vi "Beam Permit Main.vi"() -> ()   [LabVIEW 2019]
panel:
  in  "Warning sound":bool
  in  "Bypass the FMag status":bool
  out "Beam Permit":bool
  in  "Force ON Beam permit":bool
  in  "Force OFF Beam permit":bool
  out "Beam permit status":string
  out "Warning play time":u32
  out "TCP":bool
  in  "Exit VI":bool
  out "Fmag Low Current attemps":i32
  out "Error status":T1(ring)
  out "FMag monitor":u8(slide) scale=0.0..25.0
  out "chart_temp 2":waveform(dbl)[](graph)=[{"t0"=timestamp(3772890114.31303 s since 1904-01-01), "dt"=1.0, "Y"=[0.8687935985565186]}, {"t0"=timestamp(3772890114.31303 s since 1904-01-01), "dt"=1.0, "Y"=[86.87935985565186]}, {"t0"=timestamp(3772890114.31303 s since 1904-01-01), "dt"=1.0, "Y"=[30.48853325313992]}, {"t0"=timestamp(3772890114.31303 s since 1904-01-01), "dt"=1.0, "Y"=[303.6385332531399]}] caption="FMag Current"
  out "FMag Current (A)":dbl
  out "error out":errorcluster
  out "Target  Ready":bool
  out "FMag Ready":bool
  # "SpinQuest Beam Permit Signaller"
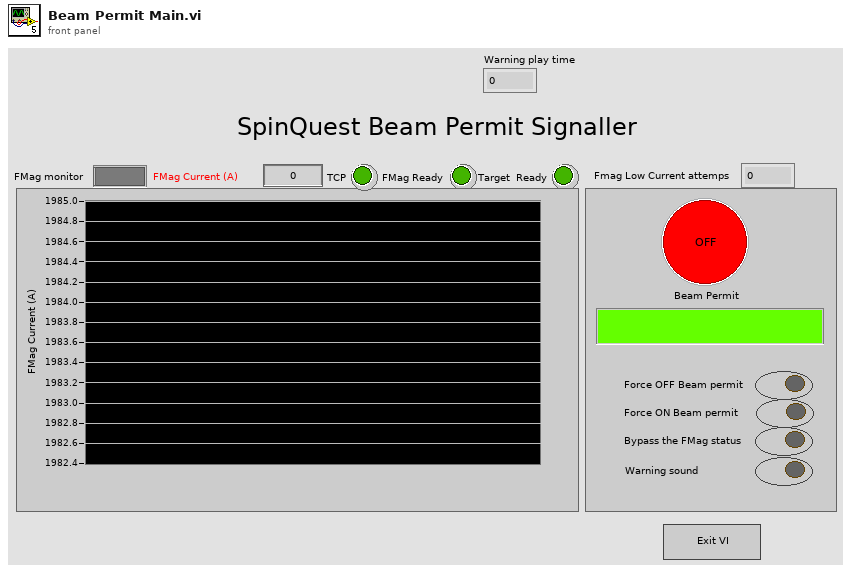
[diagram p1: front panel]
types:
  T1 = enum16{"No Error", "Les than 1800", "Les than 1500", "Les than 200", "Read out Error"}
  T2 = typedef "Sound Output Task ID.ctl" = u32
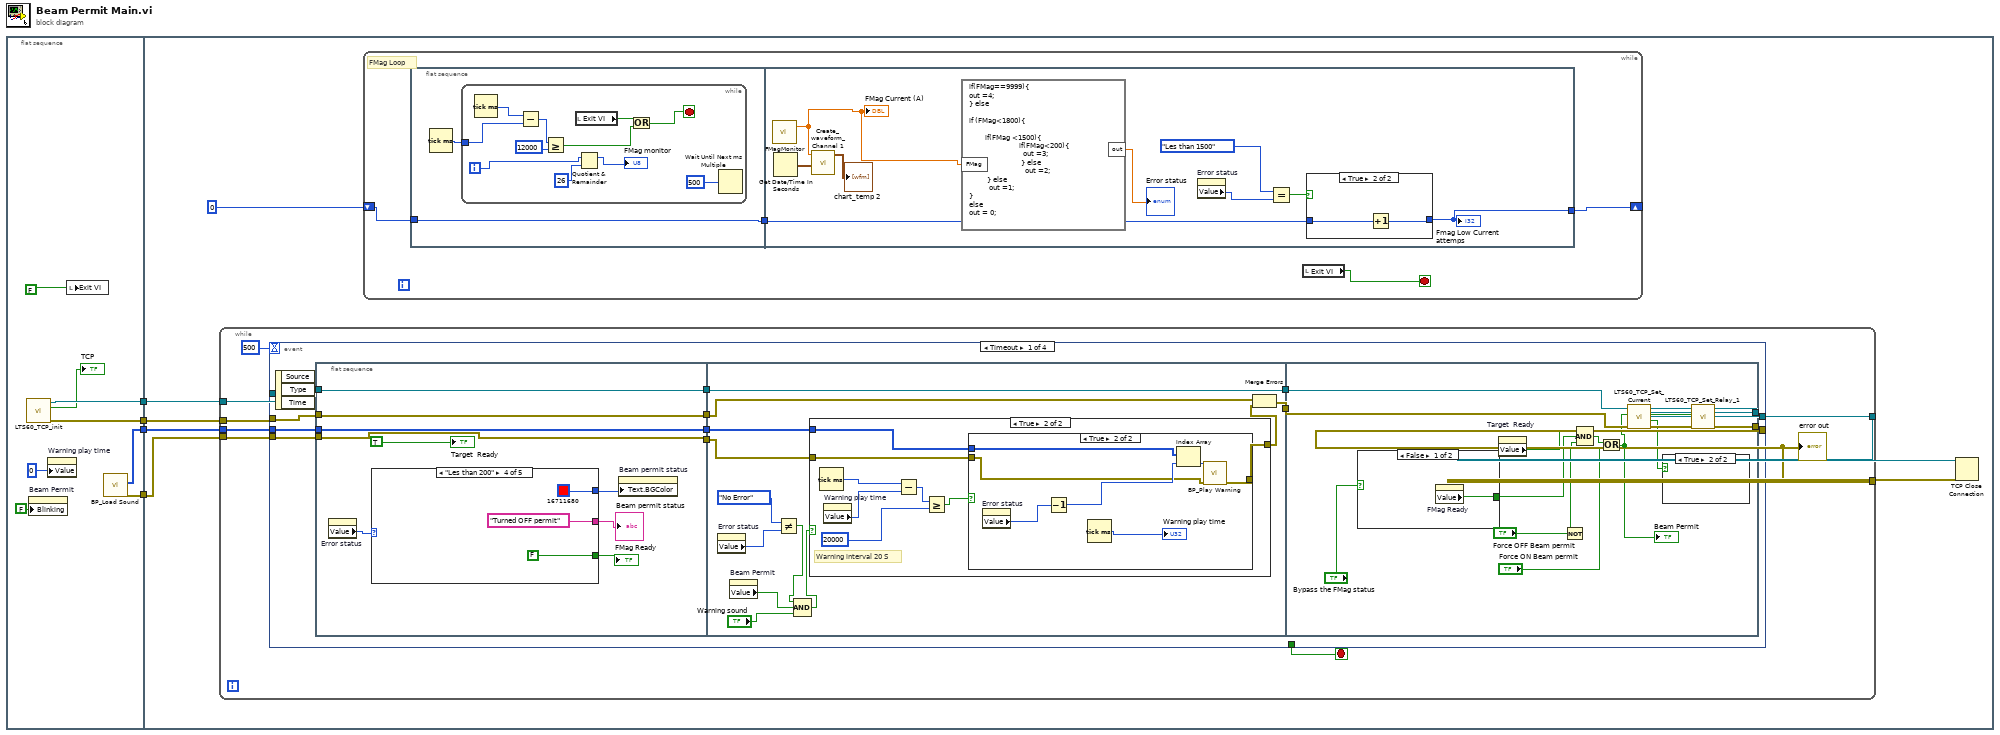
[diagram p0: block diagram]
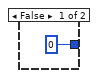
[diagram p2: hidden frame]
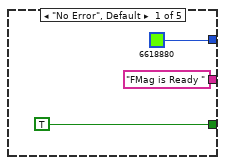
[diagram p3: hidden frame]
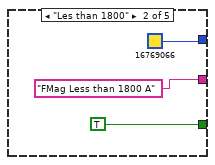
[diagram p4: hidden frame]
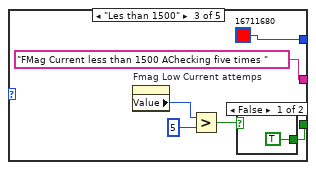
[diagram p5: hidden frame]
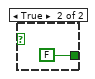
[diagram p6: hidden frame]
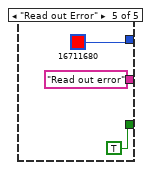
[diagram p7: hidden frame]
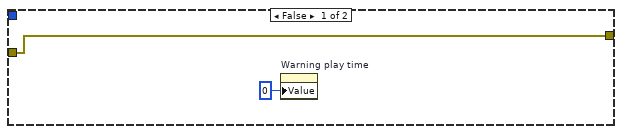
[diagram p8: hidden frame]
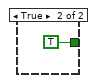
[diagram p11: hidden frame]
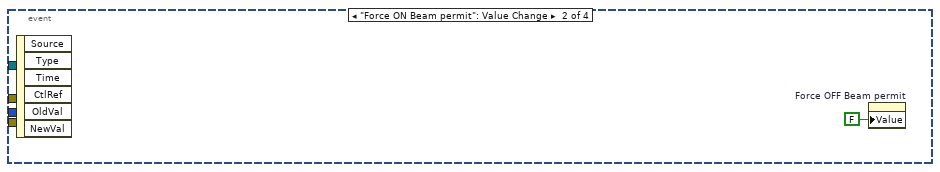
[diagram p12: hidden frame]
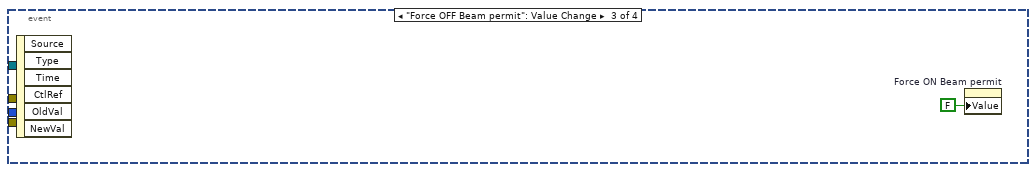
[diagram p13: hidden frame]
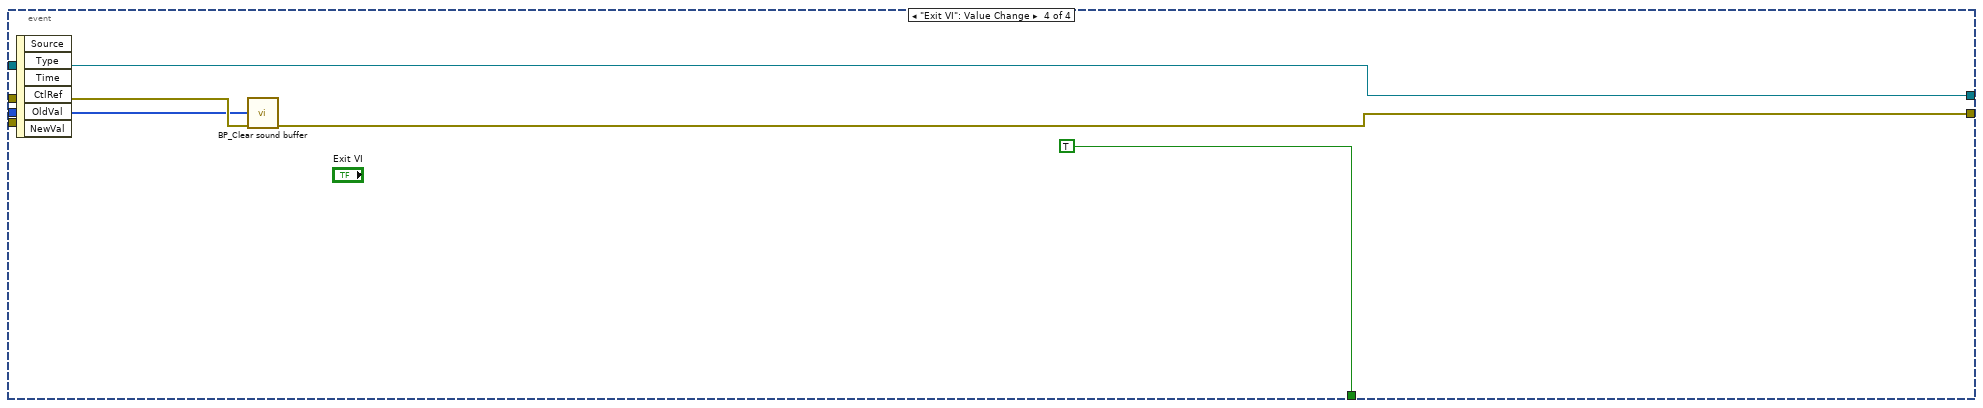
[diagram p14: hidden frame]
diagram:
  n1 = flat-sequence {
    tunnel: [w12] -> w4
    tunnel: [w11] -> w3
    tunnel: [w7] -> w2
    tunnel: [w5] -> w1
    tunnel: w4 -> [w14]
    tunnel: w3 -> [w17]
    tunnel: w2 -> [w15]
    tunnel: w1 -> [w13]
    frame #0 {
      n2 = call "LTS60_TCP_init.vi"() -> ("error out"=w12:errorcluster, "TCP Connected"=→"TCP":bool, "connection ID out"=w11:refnum<k5>)  [unwired: 9 in]
      n3 = property on="Beam Permit" class="Bool (strict)"("Blinking"=FALSE) -> ()  [unwired: 2 in, 2 out]
      n4 = property on="Warning play time" class="DigNum (strict)"("Value"=u32 0 ("Warning play time")) -> ()  [unwired: 2 in, 2 out]
      n5 = local write "Exit VI"(FALSE ("Exit VI")) -> ()
      n6 = call "BP_Load Sound.vi"() -> ("error out"=w5:errorcluster, "Sound Array"=w7:T2[])  [unwired: 9 in, 1 out]
    }
    frame #1 {
      n7 = while {
        tunnel: [w54] -> w18
        tunnel: [w53] -> w19
        tunnel: w14 -> [w52]
        tunnel: w17 -> [w51]
        tunnel: w15 -> [w50]
        tunnel: w13 -> [w49]
        stop <- w56 stop-if-true
        n8 = event shown="[0] Timeout" {
          selector: _ -> [_ _ _ _]
          dyn-events: _ -> [_ _ _ _]
          timeout: 500 -> [_ _ _ _]
          tunnel: [_ _ _ TRUE] -> w56
          tunnel: [w68 _ _ w148] -> w54
          tunnel: [w67 _ _ w151] -> w53
          tunnel: w51 -> [w65 _ _ w151]
          tunnel: w52 -> [w62 _ _ w150]
          tunnel: w50 -> [w60 _ _ w149]
          tunnel: w49 -> [w57 _ _ _]
          event Timeout {
            n9 = event-data() -> ()  [unwired: 1 in, 3 out]
            n10 = flat-sequence {
              tunnel: [w76] -> w66
              tunnel: w65 -> [w76]
              tunnel: [w75] -> w63
              tunnel: w62 -> [w75]
              tunnel: w60 -> [w71]
              tunnel: [w71] -> w59
              tunnel: [w70] -> w58
              tunnel: w57 -> [w70]
              tunnel: w66 -> [w109]
              tunnel: [w109] -> w64
              tunnel: w63 -> [w98]
              tunnel: [w100] -> w61
              tunnel: w59 -> [w106]
              tunnel: w58 -> [w101]
              tunnel: [w139] -> w68
              tunnel: [w138] -> w67
              tunnel: w64 -> [w142]
              tunnel: w61 -> [w136]
              frame #0 {
                n11 = property on="Error status" class="Enum (strict)"() -> ("Value"=w72:T1)  [unwired: 2 in, 2 out]
                n12 = case shown="\"Les than 200\"" w72 {
                  tunnel: [TRUE ("Magnet status") TRUE ("Magnet status") w89 FALSE ("Magnet status") TRUE ("Magnet status")] -> w73
                  tunnel: ["FMag is Ready " ("Beam permit status") "FMag Less than 1800 A" ("Beam permit status") "FMag Current less than 1500 AChecking five times " ("Beam permit status") "Turned OFF permit" ("Beam permit status") "Read out error" ("Beam permit status")] -> w74
                  tunnel: [u32 6618880 ("Text.Text Colors:BG Color") u32 16769066 ("Text.Text Colors:BG Color") u32 16711680 ("Text.Text Colors:BG Color") u32 16711680 ("Text.Text Colors:BG Color") u32 16711680 ("Text.Text Colors:BG Color")] -> w69
                  frame "No Error", Default {
                  }
                  frame "Les than 1800" {
                  }
                  frame "Les than 1500" {
                    n13 = property on="Fmag Low Current attemps" class="DigNum (strict)"() -> ("Value"=w88:i32)  [unwired: 2 in, 2 out]
                    n14 = Greater?(x=w88, y=5) -> (0:w86:bool)
                    n15 = case shown="False" w86 {
                      tunnel: [TRUE ("Magnet status") FALSE ("Magnet status")] -> w89
                      frame False {
                      }
                      frame True {
                      }
                    }
                  }
                  frame "Les than 200" {
                  }
                  frame "Read out Error" {
                  }
                }
                "FMag Ready" <- w73
                "Beam permit status" <- w74
                n16 = property on="Beam permit status" class="Str"("Text.BGColor"=w69) -> ()  [unwired: 2 in, 2 out]
                "Target  Ready" <- TRUE ("Target  status")
              }
              frame #1 {
                n17 = property on="Error status" class="Enum (strict)"() -> ("Value"=w108:T1)  [unwired: 2 in, 2 out]
                n18 = property on="Beam Permit" class="Bool (strict)"() -> ("Value"=w104:bool)  [unwired: 2 in, 2 out]
                n19 = Not Equal?(x=T1."No Error", y=w108) -> (x != y?=w103:bool)
                n20 = Compound Arithmetic op=AND(w103, w104, "Warning sound") -> (w102:bool)
                n21 = case shown="True" w102 {
                  tunnel: w106 -> [_ w114]
                  tunnel: [w110 w113] -> w99
                  tunnel: w101 -> [w110 w112]
                  frame False {
                    n22 = property on="Warning play time" class="DigNum (strict)"("Value"=u32 0 ("Warning play time")) -> ()  [unwired: 2 in, 2 out]
                  }
                  frame True {
                    # "Warning interval 20 S"
                    n23 = Tick Count (ms)() -> (millisecond timer value=w119:u32)
                    n24 = property on="Warning play time" class="DigNum (strict)"() -> ("Value"=w118:u32)  [unwired: 2 in, 2 out]
                    n25 = Subtract(x=w119, y=w118) -> (x-y=w117:u32)
                    n26 = Greater Or Equal?(x=w117, y=u32 20000) -> (x >= y?=w115:bool)
                    n27 = case shown="True" w115 {
                      tunnel: w114 -> [_ w125]
                      tunnel: [w120 w122] -> w113
                      tunnel: w112 -> [w120 w121]
                      frame False {
                      }
                      frame True {
                        n28 = property on="Error status" class="Enum (strict)"() -> ("Value"=w127:T1)  [unwired: 2 in, 2 out]
                        n29 = Decrement(x=w127) -> (x-1=w124:T1)
                        n30 = Tick Count (ms)() -> (millisecond timer value=→"Warning play time":u32)
                        n31 = Index Array(array=w125, index=w124) -> (element=w123:T2)
                        n32 = call "BP_Play Warning.vi"("error in (no error)"=w121, "task ID"=w123) -> ("error out"=w122:errorcluster)  [unwired: 8 in, 1 out]
                      }
                    }
                  }
                }
                n33 = Merge Errors(w98, w99) -> (w100:errorcluster)
              }
              frame #2 {
                n34 = case shown="False" "Bypass the FMag status" {
                  tunnel: [w144 TRUE ("Value")] -> w132
                  frame False {
                    n35 = property on="FMag Ready" class="Bool (strict)"() -> ("Value"=w144:bool)  [unwired: 2 in, 2 out]
                  }
                  frame True {
                  }
                }
                n36 = property on="Target  Ready" class="Bool (strict)"() -> ("Value"=w143:bool)  [unwired: 2 in, 2 out]
                n37 = Not(x="Force OFF Beam permit") -> (.not. x?=w131:bool)
                n38 = Compound Arithmetic op=AND(w143, w132, w131) -> (w134:bool)
                n39 = Or(x=w134, y="Force ON Beam permit") -> (x .or. y?=w129:bool)
                "Beam Permit" <- w129
                n40 = call "LTS60_TCP_Set_Current.vi"("error in (no error)"=w136, "Beam"=w129, "connection ID"=w142) -> ("error out"=w140:errorcluster, "Acknowladged"=w128:bool, "Beam out"=w137:bool, "connection ID out"=w141:refnum<k5>)  [unwired: 5 in]
                n41 = case shown="True" w128 {
                  frame False {
                  }
                  frame True {
                  }
                }
                n42 = call "LTS60_TCP_Set_Relay_1.vi"("error in (no error)"=w140, "Beam"=w137, "connection ID"=w141) -> ("error out"=w139:errorcluster, "connection ID out"=w138:refnum<k5>)  [unwired: 6 in, 1 out]
              }
            }
          }
          event "Force ON Beam permit": Value Change {
            n43 = event-data() -> ()  [unwired: 1 in, 6 out]
            n44 = property on="Force OFF Beam permit" class="Bool (strict)"("Value"=FALSE ("Force OFF Beam permit")) -> ()  [unwired: 2 in, 2 out]
          }
          event "Force OFF Beam permit": Value Change {
            n45 = event-data() -> ()  [unwired: 1 in, 6 out]
            n46 = property on="Force ON Beam permit" class="Bool (strict)"("Value"=FALSE ("Force ON Beam permit")) -> ()  [unwired: 2 in, 2 out]
          }
          event "Exit VI": Value Change {
            n47 = event-data() -> ()  [unwired: 1 in, 6 out]
            n48 = call "BP_Clear sound buffer.vi"("error in (no error)"=w150, "array"=w149) -> ("error out"=w148:errorcluster)  [unwired: 9 in]
          }
        }
        "error out" <- w54
      }
      n49 = while {
        shift-right: [w21] -> _
        shift-left: 0 ("Low Fmag attemps") -> [w23]
        stop <- w20 stop-if-true
        # "FMag Loop"
        n50 = flat-sequence {
          tunnel: w23 -> [w24]
          tunnel: [w24] -> w22
          tunnel: w22 -> [w41]
          tunnel: [w40] -> w21
          frame #0 {
            n51 = Tick Count (ms)() -> (millisecond timer value=w25:u32)
            n52 = while {
              tunnel: w25 -> [w34]
              i -> [w29]
              stop <- w27 stop-if-true
              n53 = Tick Count (ms)() -> (millisecond timer value=w35:u32)
              n54 = Subtract(x=w35, y=w34) -> (x-y=w33:u32)
              n55 = Greater Or Equal?(x=w33, y=u32 12000) -> (x >= y?=w26:bool)
              n56 = local read "Exit VI"() -> (w28:bool)
              n57 = Quotient & Remainder(x=w29, y=u32 26) -> (x-y*floor(x/y)=→"FMag monitor":u32)  [unwired: 1 out]
              n58 = Or(x=w28, y=w26) -> (x .or. y?=w27:bool)
              n59 = Wait Until Next ms Multiple(millisecond multiple=u32 500) -> ()  [unwired: 1 out]
            }
          }
          frame #1 {
            n60 = call "FMagMonitor.vi"() -> ("FMag Current"=w37:dbl)  [unwired: 2 in, 1 out]
            "FMag Current (A)" <- w37
            n61 = Get Date/Time In Seconds() -> (seconds since 1Jan1904=w45:timestamp)
            n62 = call "Create_waveform_Channel 1.vi"("time"=w45, "Channel 1"=w37) -> ("waveform_array"=→"chart_temp 2":waveform(dbl)[])  [unwired: 9 in]
            n63 = formula code="if(FMag==9999){\nout =4;\n} else\n\nif (FMag<1800){\n       \n        if(FMag <1500){\n                         if(FMag<200){\n                           out =3;\n                          } else \n                            out =2;\n         } else\n          out =1;\n}\nelse\nout = 0;"("FMag"=w37) -> ("out"=→"Error status":dbl)
            n64 = property on="Error status" class="Enum (strict)"() -> ("Value"=w39:T1)  [unwired: 2 in, 2 out]
            n65 = Equal?(x=T1."Les than 1500", y=w39) -> (x = y?=w42:bool)
            n66 = case shown="True" w42 {
              tunnel: [0 ("Low Fmag attemps") w48] -> w40
              tunnel: w41 -> [_ w47]
              frame False {
              }
              frame True {
                n67 = Increment(x=w47) -> (x+1=w48:i32)
              }
            }
            "Fmag Low Current attemps" <- w40
          }
        }
        n68 = local read "Exit VI"() -> (w20:bool)
      }
      n69 = TCP Close Connection(connection ID=w19, error in (no error)=w18) -> ()  [unwired: 1 in, 2 out]
    }
  }
